vi "DHE_GetAsyncN.vi"() -> (2 "asyncN":refnum<notifier>)   [LabVIEW 2016]
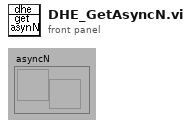
[diagram p1: front panel]
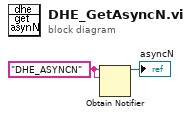
[diagram p0: block diagram]
diagram:
  w2 = "DHE_ASYNCN" ("name (unnamed)")
  n1 = Obtain Notifier(name (unnamed)=w2, notification data type=w2) -> (notifier out=→"asyncN":refnum<notifier>)  [unwired: 2 in, 2 out]
